vi "4_1_PTLF_Classification_Inference(CPU,GPU,RT).vi"() -> ()   [LabVIEW 2020]
uses:
  <vilib>/Ngene/Deep Learning Toolkit/Toolkit/NN_Network/Controls/NN_Device.ctl
  <vilib>/Ngene/Deep Learning Toolkit/Toolkit/NN_Network/Controls/NN_Save_Before_Destroy_Options.ctl
  <vilib>/Ngene/Deep Learning Toolkit/Toolkit/NN_Network/API/NN_Set_Input/1D/NN_Set_Input(1D_SGL_idx).vi
  <vilib>/Ngene/Deep Learning Toolkit/Toolkit/Deep_Learning_Toolkit_by_Ngene.lvlib
  <vilib>/measure/NI_MABase.lvlib
  <vilib>/ptbypt/NI_PtbyPt.lvlib
panel:
  in  "NN_Device":T1
  out "error out":errorcluster
  out "Inference Time":dbl=0.000547710000000734 format="%#_3p"
  out "Loop Time":dbl=0.0006916499999988446 format="%#_3p"
  in  "Position":dbl(slide)=0.4116719242902208 scale=0.0..1.0
  in  "Fault Generation":T2(tab)=enum."Swell"
  in  "scale":sgl(slide)=0.6375 scale=0.5..0.7
  in  "Duration(#s)":i32(slide)=388 scale=200.0..600.0
  in  "scale":sgl(slide)=1.4484375 scale=1.35..1.5
  in  "Duration(#s)":i32(slide)=458 scale=200.0..600.0
  in  "Duration(#s)":i32(slide)=366 scale=200.0..600.0
  in  "Tau":dbl(slide)=337.5 scale=200.0..600.0
  in  "Frequency":dbl(slide)=1666.6666666666665 scale=1000.0..2000.0
  in  "Amplitude":dbl(slide)=184.375 scale=150.0..200.0
  in  "Offset":sgl(slide)=105.208336 scale=50.0..150.0
  in  "Duration(#s)":i32(slide)=449 scale=200.0..600.0
  out "Predicted Class":string="Swell"
  out "Class Labels":string[](array[string])=["DC Offset", "Interruption", "Normal", "Sag", "Swell", "Transient"]
  out "Generated WaveForm":waveform(sgl)(graph)={"t0"=timestamp(0 s since 1904-01-01), "dt"=1.0, "Y"=array[2000 elements]}
  in  "Weight File Path":path=path "D:/Ngene/GitHub/deepltk_fpga_examples/3_PTLF_Classification(PXI,sbRIO)/Models/0_PTLF_Classification_Original/PTLF_Classifier_weights_24_11_21__13_37_15.bin"
  in  "Configuration File Path":path=path "D:/Ngene/GitHub/deepltk_fpga_examples/3_PTLF_Classification(PXI,sbRIO)/Models/0_PTLF_Classification_Original/PTLF_Classifier_net_cfg_24_11_21__13_37_15.cfg"
  out "Class Probabilities":sgl[](array[slide])=[7.445699e-08, 1.3515468e-05, 1.2787451e-09, 0.0016558456, 0.9983304, 1.4073053e-07] scale=0.0..1.0
  in  "Stop":bool
  # "Overview: Demonstrates the usage of Deep Learning Toolkit for loading the model pretrained for Power Line Fault Classification and running for inference on CPU or GPU.\nRequirements: \n• DeepLTK - Deep Learning Toolkit for LabVIEW (https://www.ngene.co/deep-learning-toolkit-for-labview)\nInstructions:\nNote: To run the example on an RT target, copy the pretrained model to the RT target.\n1.\tProvide the \"Configuration File Path\" and \"Weight File Path\" generated by 1_PTLF_Classification_Training.vi or sample from project (located in \"Models\\1_PTLF_Classification_Original\" folder.\n2.\tUse NN_Device to specify the device (CPU or GPU) for execution. GPU is applicable only for 64-bit LabVIEW.\n3.\tRun the VI.\n4. Choose type of the fault and change the parameters and observe the predicted type of the fault.\n5. Press the Stop button to stop the VI.\nMore Examples: https://github.com/ngenehub/deepltk_fpga_examples"
  # "Power Transmission Line Fault Classification - Inference on CPU"
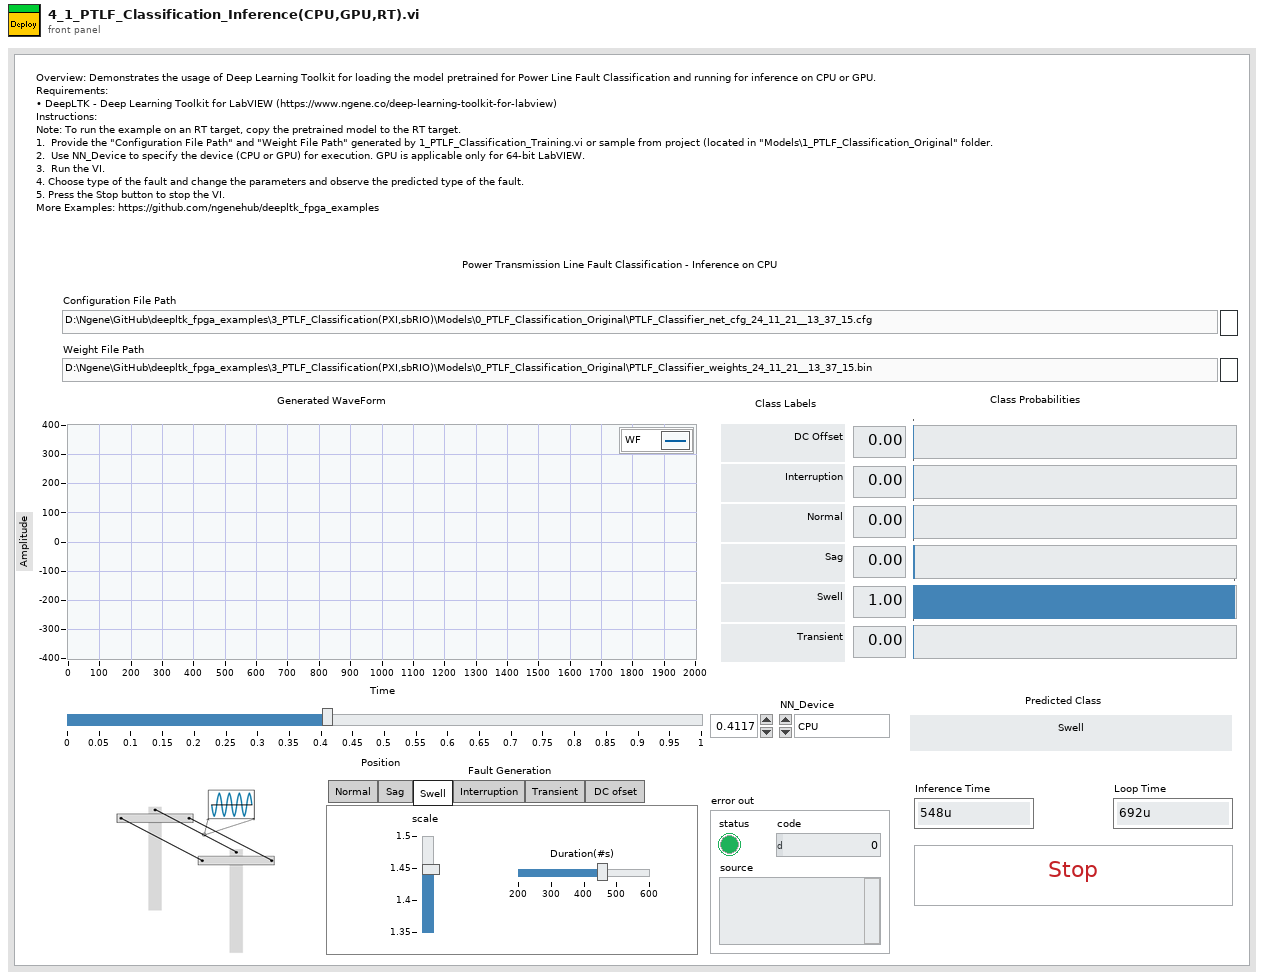
[diagram p1: front panel]
types:
  T1 = typedef "Deep_Learning_Toolkit_by_Ngene.lvlib/NN_Device.ctl" = enum16{"CPU", "GPU"}
  T2 = enum32{"Normal", "Sag ", "Swell", "Interruption", "Transient", "DC ofset "}
  T3 = typedef "Deep_Learning_Toolkit_by_Ngene.lvlib/NN_Save_Before_Destroy_Options.ctl" = cluster{"CFG?":bool, "Weights?":bool, "Render?":bool}
  T4 = typedef "Deep_Learning_Toolkit_by_Ngene.lvlib/NN_Config_Params.ctl" = cluster{"Name":string, "mBatch":i32, "NN_Train_Params":T5, "LR_Decay_Policy":T8, "Labels":string[], "Loss":T10}
  T5 = typedef "Deep_Learning_Toolkit_by_Ngene.lvlib/NN_Train_Params.ctl" = cluster{"Optimizer":T6, "Beta_1":sgl, "Beta_2":sgl, "Weight Decay(L1)":sgl, "Weight Decay(L2)":sgl, "Data_Sampling":T7}
  T6 = typedef "Deep_Learning_Toolkit_by_Ngene.lvlib/NN_Train_Optimizer.ctl" = enum16{"SGD", "Adam", "Adagrad", "Adadelta", "RMSProp", "Nesterov"}
  T7 = typedef "Deep_Learning_Toolkit_by_Ngene.lvlib/NN_Train_Data_Sampling.ctl" = enum16{"Random", "Sequential"}
  T8 = typedef "Deep_Learning_Toolkit_by_Ngene.lvlib/NN_LR_Policy_Cfg.ctl" = cluster{"Policy_Type":T9, "LR0":dbl, "k":sgl, "WarmUp_Policy":enum16{"Step", "Ramp"}, "WarmUp_Iter":i32, "WarmUp_Ratio":sgl}
  T9 = typedef "Deep_Learning_Toolkit_by_Ngene.lvlib/NN_LR_Policy_Type.ctl" = enum16{"Manual", "Step", "Exp", "1/t"}
  T10 = typedef "Deep_Learning_Toolkit_by_Ngene.lvlib/NN_Loss_Config_Params.ctl" = cluster{"Loss_Type":T11, "Loss_Conf_Params":variant}
  T11 = typedef "Deep_Learning_Toolkit_by_Ngene.lvlib/NN_Loss_Type.ctl" = enum16{"None", "MSE", "CrossEntropy", "YOLO_v2", "YOLO_v4"}
  T12 = typedef "Deep_Learning_Toolkit_by_Ngene.lvlib/NN_Layer_Config_Params.ctl" = cluster{"Layer_Type":T13, "Layer_Conf_Params":variant, "Input Layers":string[]}
  T13 = typedef "Deep_Learning_Toolkit_by_Ngene.lvlib/NN_Layer_Type.ctl" = enum16{"Input1D", "Input3D", "Conv1D", "Conv2D", "Conv2D_Adv", "MaxPool", "AvgPool", "UpSample", "DropOut3D", "ShortCut", "Concat", "SoftMax3D", "FC", "DropOut", "Softmax", "Flatten", "YOLO_v2", "YOLO_v4", "Activation", "BatchNormalization", "Unsupported"}
  T14 = typedef "Deep_Learning_Toolkit_by_Ngene.lvlib/NN.ctl" = cluster{"Name":string, "No of Layers":i32, "mBatch":i32, "Layers":T15[], "Dimty":T16, "Dims_In":T17, "Dims_Out":T17, "Working_Dir":path, "Train?":bool, "Train_Params":T5, "LR_Update_Policy":T8, "Session Data":T18, "Ground_truth":T19, "NNg_hdls":T20, "NN_Device":T1, "GPU Id":i32, "Labels":string[], "Receptive Field":T21[], "Loss_Type":T11, "Loss_Cfg_Prms":variant, "NNG_WS":T22}
  T15 = typedef "Deep_Learning_Toolkit_by_Ngene.lvlib/NN_Layer_ref.ctl" = refnum<data-value>
  T16 = typedef "Deep_Learning_Toolkit_by_Ngene.lvlib/NN_In_Out_Dim-ty.ctl" = enum8{"In1D_Out1D", "In3D_Out1D", "In3D_Out3D", "In3D_OutBBox"}
  T17 = typedef "Deep_Learning_Toolkit_by_Ngene.lvlib/NN_Dims(C,H,W).ctl" = cluster{"C":i32, "H":i32, "W":i32}
  T18 = typedef "Deep_Learning_Toolkit_by_Ngene.lvlib/NN_Train_Session_Data.ctl" = cluster{"Epochs":sgl, "Tot_Iter":i32, "LR":sgl, "LR_iter":i32}
  T19 = typedef "Deep_Learning_Toolkit_by_Ngene.lvlib/NN_Ground_truth.ctl" = cluster{"Y":variant}
  T20 = typedef "Deep_Learning_Toolkit_by_Ngene.lvlib/nng_cuda_handles.ctl" = cluster{"cudnn":u64, "cublas":u64, "stream":u64, "curand":u64}
  T21 = typedef "Deep_Learning_Toolkit_by_Ngene.lvlib/NN_Dims(V,H).ctl" = cluster{"V":i32, "H":i32}
  T22 = typedef "Deep_Learning_Toolkit_by_Ngene.lvlib/NNG_WS.ctl" = cluster{"NNG_WS_Mem":T23, "Max_WS_Size":i64}
  T23 = typedef "Deep_Learning_Toolkit_by_Ngene.lvlib/NNg_WS_Mem_DVR.ctl" = refnum<data-value>
  T24 = typedef "Deep_Learning_Toolkit_by_Ngene.lvlib/NN_Layer.ctl" = cluster{"Name":string, "Layer_Data":variant, "Layer_Type":T13, "Dims_In":T17, "Layers_In":variant, "Dims_Out":T17, "Layers_Out":variant, "Metrics":T25, "GPU_Data":variant, "mBatch":i32, "NN_Device":T1, "NNg_hdls":T20, "Train?":bool, "Dimty":T26, "RecptField":T27}
  T25 = typedef "Deep_Learning_Toolkit_by_Ngene.lvlib/NN_Layer_Metrics.ctl" = cluster{"Data":dbl, "Params":dbl, "Ops":dbl}
  T26 = typedef "Deep_Learning_Toolkit_by_Ngene.lvlib/NN_Layer_Dimty.ctl" = enum16{"1D", "3D"}
  T27 = typedef "Deep_Learning_Toolkit_by_Ngene.lvlib/NN_Layer_RF_State.ctl" = cluster{"Dims":T21, "J":T21}
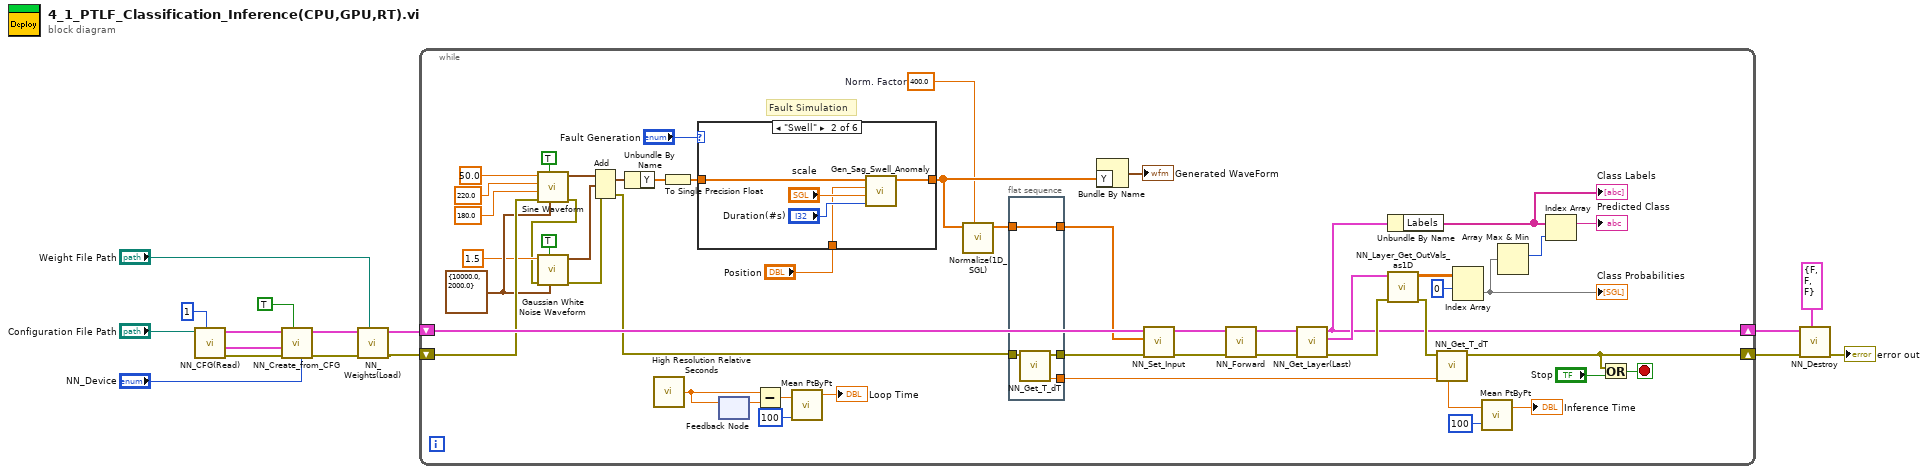
[diagram p0: block diagram]
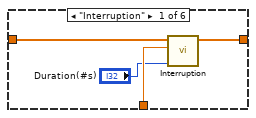
[diagram p2: hidden frame]
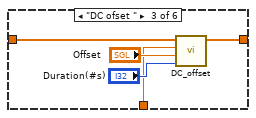
[diagram p3: hidden frame]
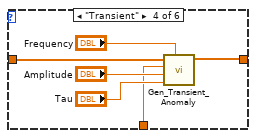
[diagram p4: hidden frame]
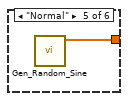
[diagram p5: hidden frame]
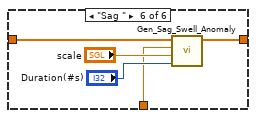
[diagram p6: hidden frame]
diagram:
  n1 = call <vilib>:"NN_CFG(Read).vi"("mBatch"=1, "CFG file path"="Configuration File Path") -> ("error out"=w13:errorcluster, "Net_Cfg"=w11:T4, "Layer_Cfg"=w8:T12[])  [unwired: 7 in]
  n2 = call <vilib>:"NN_Create_from_CFG.vi"("NN_Device"="NN_Device", "Train? (false)"=TRUE, "error in (no error)"=w13, "Net_Cfg"=w11, "Layer_Cfg"=w8) -> ("error out"=w12:errorcluster, "NN out"=w7:T14)  [unwired: 5 in]
  n3 = call <vilib>:"NN_Weights(Load).vi"("Weight File Path"="Weight File Path", "error in (no error)"=w12, "NN in"=w7) -> ("error out"=w5:errorcluster, "NN out"=w6:T14)  [unwired: 7 in]
  n4 = while {
    shift-right: [w27] -> w16
    shift-left: w5 -> [w48]
    shift-right: [w18] -> w15
    shift-left: w6 -> [w61]
    stop <- w28 stop-if-true
    w35 = sgl 400.0  # Norm. Factor
    w46 = cluster{"Fs":dbl, "#s":dbl} {"Fs"=10000.0, "#s"=2000.0} ("sampling info")
    # "Fault Simulation"
    n5 = call <vilib>:"Sine Waveform.vi"("sampling info"=w46, "reset signal"=TRUE, "error in (no error)"=w48, "phase"=180.0, "amplitude"=220.0, "frequency"=50.0) -> ("error out"=w42:errorcluster, "signal out"=w56:waveform(dbl))  [unwired: 4 in]
    n6 = call <vilib>:"Gaussian White Noise Waveform.vi"("sampling info"=w46, "reset signal"=TRUE, "error in (no error)"=w42, "standard deviation"=sgl 1.5 ("Noise Standart Deviation")) -> ("error out"=w41:errorcluster, "signal out"=w34:waveform(dbl))  [unwired: 6 in]
    n7 = Add(1:w34, 2:w56, 4:w41) -> (0:w44:waveform(dbl), 3:w30:errorcluster)
    n8 = Unbundle By Name(w44) -> ("Y"=w55:dbl[])
    n9 = call <vilib>:"High Resolution Relative Seconds.vi"() -> ("relative seconds"=w36:dbl)
    n10 = To Single Precision Float(number=w55) -> (single precision float=w52:sgl[])
    n11 = case shown="\"Swell\"" "Fault Generation" {
      tunnel: [w74 w77 w82 w90 w92 w94] -> w40
      tunnel: w52 -> [w75 w80 w85 w91 _ w97]
      tunnel: "Position" -> [w73 w76 w81 w86 _ w93]
      frame "Interruption" {
        n12 = call "Interruption.vi"("Duration"="Duration(#s)", "Position"=w73, "Sine"=w75) -> ("Sine+Anomaly"=w74:sgl[])  [unwired: 8 in]
      }
      frame "Swell" {
        n13 = call "Gen_Sag_Swell_Anomaly.vi"("Duration"="Duration(#s)", "Amplitude"="scale", "Position"=w76, "Sine"=w80) -> ("Sine+Anomaly"=w77:sgl[])  [unwired: 7 in]
      }
      frame "DC ofset " {
        n14 = call "DC_offset.vi"("Duration"="Duration(#s)", "Ampltude"="Offset", "Position"=w81, "Sine"=w85) -> ("Sine+Anomaly"=w82:sgl[])  [unwired: 7 in]
      }
      frame "Transient" {
        n15 = call "Gen_Transient_Anomaly.vi"("Frequency"="Frequency", "Tau"="Tau", "Amplitude"="Amplitude", "Position"=w86, "Sine"=w91) -> ("Sine+Anomaly"=w90:sgl[])  [unwired: 6 in]
      }
      frame "Normal" {
        n16 = call "Gen_Random_Sine.vi"() -> ("data"=w92:sgl[])  [unwired: 11 in]
      }
      frame "Sag " {
        n17 = call "Gen_Sag_Swell_Anomaly.vi"("Duration"="Duration(#s)", "Amplitude"="scale", "Position"=w93, "Sine"=w97) -> ("Sine+Anomaly"=w94:sgl[])  [unwired: 7 in]
      }
    }
    n18 = feedback #1() -> (w37:dbl)  [unwired: 1 in]
    n19 = feedback-in #1(w36) -> ()
    n20 = Subtract(x=w36, y=w37) -> (x-y=w39:dbl)
    n21 = call <vilib>:"Mean PtByPt.vi"("x"=w39, "sample length"=100) -> ("mean"=→"Loop Time":dbl)  [unwired: 2 in, 1 out]
    n22 = call "Normalize(1D_SGL).vi"("Norm. Factor"=w35, "Data In"=w40) -> ("Normalized Out"=w25:sgl[])  [unwired: 9 in]
    n23 = flat-sequence {
      tunnel: [w71] -> w33
      tunnel: [w70] -> w31
      tunnel: w30 -> [w69]
      tunnel: w25 -> [w68]
      tunnel: [w68] -> w24
      frame #0 {
        n24 = call <vilib>:"NN_Get_T_dT.vi"("error in (no error)"=w69) -> ("T_out"=w70:dbl, "error out"=w71:errorcluster)  [unwired: 6 in, 1 out]
      }
    }
    n25 = Bundle By Name("Y"=w40) -> (→"Generated WaveForm":waveform(sgl))  [unwired: 1 in]
    n26 = call-poly <vilib>:"NN_Set_Input.vi"("error in (no error)"=w33, "Data_In(1D_SGL)"=w24, "NN In"=w61) -> ("error out"=w66:errorcluster, "NN Out"=w65:T14)  [unwired: 7 in]
    n27 = call <vilib>:"NN_Forward.vi"("error in (no error)"=w66, "NN in"=w65) -> ("error out"=w32:errorcluster, "NN out"=w20:T14)  [unwired: 6 in, 2 out]
    n28 = call <vilib>:"NN_Get_Layer(Last).vi"("error in (no error)"=w32, "NN in"=w20) -> ("error out"=w21:errorcluster, "Last_Layer"=w19:T24, "NN out"=w18:T14)  [unwired: 6 in, 1 out]
    n29 = Unbundle By Name(w18) -> ("Labels"=w17:string[])
    "Class Labels" <- w17
    n30 = call <vilib>:"NN_Layer_Get_OutVals_as1D.vi"("error in (no error)"=w21, "Layer"=w19) -> ("error out"=w67:errorcluster, "Out(as1D)"=w64:sgl[][])  [unwired: 8 in]
    n31 = call <vilib>:"NN_Get_T_dT.vi"("T_in"=w31, "error in (no error)"=w67) -> ("error out"=w27:errorcluster, "dT"=w29:dbl)  [unwired: 5 in, 1 out]
    n32 = Index Array(array=w64, index (row)=0) -> (element=w60:sgl[])  [unwired: 1 in]
    "Class Probabilities" <- w60
    n33 = call <vilib>:"Mean PtByPt.vi"("x"=w29, "sample length"=100) -> ("mean"=→"Inference Time":dbl)  [unwired: 2 in, 1 out]
    n34 = Array Max & Min(array=w60) -> (max index (indices)=w59:i32)  [unwired: 3 out]
    n35 = Index Array(array=w17, index=w59) -> (element=→"Predicted Class":string)
    n36 = Or(x=w27, y="Stop") -> (x .or. y?=w28:bool)
  }
  n37 = call <vilib>:"NN_Destroy.vi"("Save (T, T, T)"=T3 {"CFG?"=FALSE, "Weights?"=FALSE, "Render?"=FALSE}, "error in (no error)"=w16, "NN in"=w15) -> ("error out"=→"error out":errorcluster)  [unwired: 7 in, 1 out]
